vi "globalSetUp.vi"(8 "error in":errorcluster, 11 "Deployment in":refnum<class "Deployment.lvclass">) -> (0 "error out":errorcluster, 3 "Deployment out":refnum<class "Deployment.lvclass">)   [LabVIEW 2020, in "Deployment.lvclass"]
uses:
  Deployment.lvclass
  niveristand-custom-device-testing-tools/VeriStandTestUtilities/VeriStandTestUtilities.lvlib
  Scripting/Communication Bus Template Scripting.lvlib
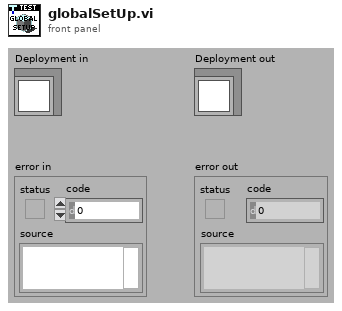
[diagram p1: front panel]
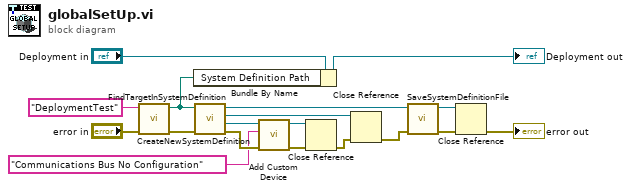
[diagram p0: block diagram]
diagram:
  n1 = call "CreateNewSystemDefinition.vi"("error in"="error in", "System Definition Name"="DeploymentTest") -> ("error out"=w12:errorcluster, "System Definition Path"=w13:path)  [unwired: 8 in]
  n2 = Bundle By Name(cluster="Deployment in", "System Definition Path"=w13) -> (→"Deployment out":refnum<class "Deployment.lvclass">)
  n3 = call "FindTargetInSystemDefinition.vi"("error in"=w12, "system definition path"=w13) -> ("error out"=w3:errorcluster, "Target"=w5:refnum<k24>, "Root"=w8:refnum<k24>, "System Definition"=w7:refnum<k24>)  [unwired: 6 in]
  n4 = call "Add Custom Device.vi"("error in"=w3, "name"="Communications Bus No Configuration", "target in"=w5) -> ("error out"=w2:errorcluster, "target out"=w4:refnum<k24>)  [unwired: 6 in, 1 out]
  n5 = Close Reference(reference=w4, error in (no error)=w2) -> (error out=w17:errorcluster)
  n6 = Close Reference(reference=w8, error in (no error)=w17) -> (error out=w18:errorcluster)
  n7 = call "SaveSystemDefinitionFile.vi"("error in (no error)"=w18, "System Definition Reference in"=w7) -> ("error out"=w16:errorcluster, "System Definition Reference out"=w15:refnum<k24>)  [unwired: 8 in]
  n8 = Close Reference(reference=w15, error in (no error)=w16) -> (error out=→"error out":errorcluster)
